vi "ReadData5.vi"() -> ()   [LabVIEW 2013]
uses:
  <vilib>/Utility/file.llb/Read From Spreadsheet File (DBL).vi
  <vilib>/Analysis/NI_AALPro.lvlib
  <vilib>/Analysis/NI_AALBase.lvlib
panel:
  out "Residual (V)":dbl format="%#_3g"
  in  "1st sweep":i32=400
  out "Peak Area Distribution":cluster{"Y":dbl[], "Y":dbl[]}[](graph)=[{"Y"=[nan, nan, nan, nan, nan, nan, nan, nan, nan, nan, nan, nan, nan, nan, nan, nan, nan, nan, nan, nan, nan, nan, nan, nan, nan, nan, nan, nan, nan, nan, nan, nan, nan, nan, nan, nan, nan, nan, nan, nan, nan, nan, nan, nan, nan, nan, nan, nan, nan, nan, nan, nan, nan, nan, nan, nan, nan, nan, nan, nan, nan, nan, nan, nan, nan, nan, nan, nan, nan, nan, nan, nan, nan, nan, nan, nan, nan, nan, nan, nan, nan, nan, nan, nan, nan, nan, nan, nan, nan, nan, nan, nan, nan, nan, nan, nan, nan, nan, nan, nan], "Y"=[0.0, 0.0, 0.0, 0.0, 0.0, 0.0, 0.0, 0.0, 0.0, 0.0, 0.0, 0.0, 0.0, 0.0, 0.0, 0.0, 0.0, 0.0, 0.0, 0.0, 0.0, 0.0, 0.0, 0.0, 0.0, 0.0, 0.0, 0.0, 0.0, 0.0, 0.0, 0.0, 0.0, 0.0, 0.0, 0.0, 0.0, 0.0, 0.0, 0.0, 0.0, 0.0, 0.0, 0.0, 0.0, 0.0, 0.0, 0.0, 0.0, 0.0, 0.0, 0.0, 0.0, 0.0, 0.0, 0.0, 0.0, 0.0, 0.0, 0.0, 0.0, 0.0, 0.0, 0.0, 0.0, 0.0, 0.0, 0.0, 0.0, 0.0, 0.0, 0.0, 0.0, 0.0, 0.0, 0.0, 0.0, 0.0, 0.0, 0.0, 0.0, 0.0, 0.0, 0.0, 0.0, 0.0, 0.0, 0.0, 0.0, 0.0, 0.0, 0.0, 0.0, 0.0, 0.0, 0.0, 0.0, 0.0, 0.0, 0.0]}]
  in  "# of sweeps":i32=500
  out "Mean Error":dbl=nan format="%#_2g"
  out "Mean Area":dbl=nan format="%#_4g"
  out "Peak Area":dbl(graph)=nan
  out "Spectrum #":i32=499
  out "Chars":i32=640716
  out "Fcen":dbl=213.0 format="%#_13g"
  in  "Fmin":dbl=212.8 format="%#_13g"
  in  "Fmax":dbl=213.2 format="%#_13g"
  out "# Data points":i32=81
  out "Peak Area (V-MHz)":dbl=nan format="%#_3g"
  out "Offset V":dbl=-0.006412499999999998 format="%#_3g"
  out "RMS Fit Error (V)":dbl=nan format="%#_2g"
  in  "Start sigma (V)":dbl=0.01 format="%#_13g"
  in  "Start offset (V)":dbl format="%#_13g"
  out "FWHM (MHz)":dbl=nan format="%#_3g"
  out "Center Freq (MHz)":dbl=nan
  out "Amplitude (V)":dbl=nan format="%#_3g"
  out "NMR Graph + Fit":cluster{cluster{dbl, "Numeric":dbl}[]}[](graph)
  out "File size (bytes)":i32=1284000
  out "File name":string="C:\\Documents and Settings\\Patrick McGaughey\\Desktop\\rssmt\\NMR3489061581.xls"
  # "Gaussian Fit Results"
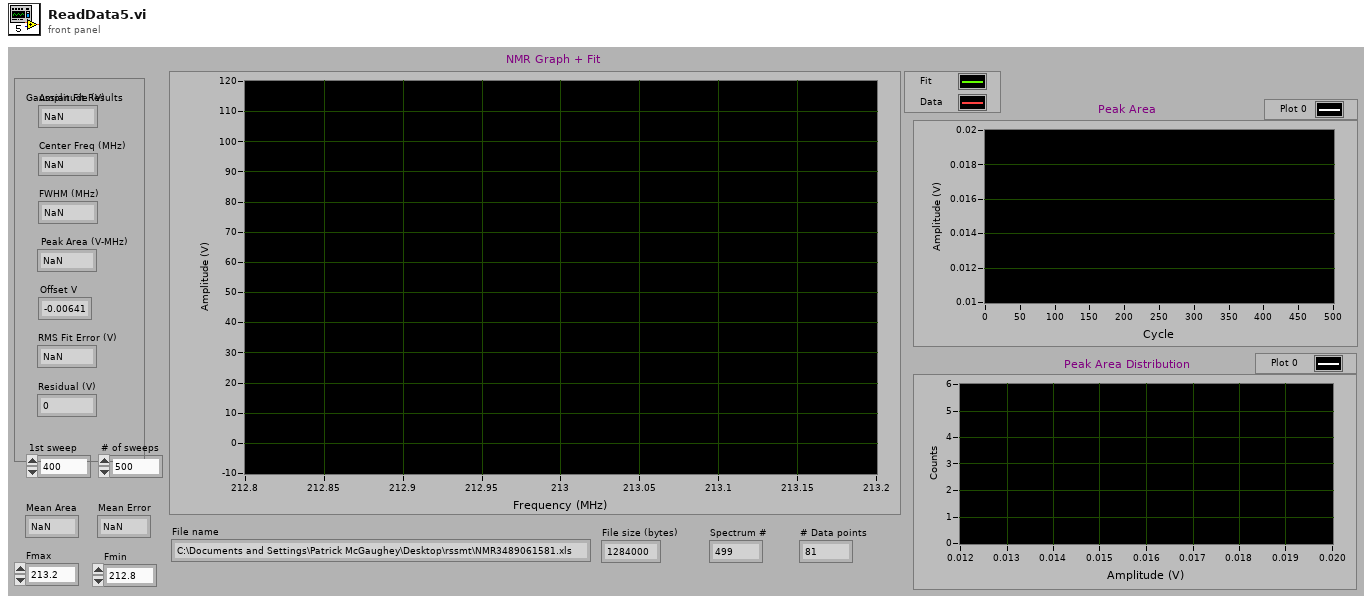
[diagram p1: front panel]
types:
  T1 = cluster{dbl, dbl, "Start sigma (V)":dbl, "Start offset (V)":dbl}
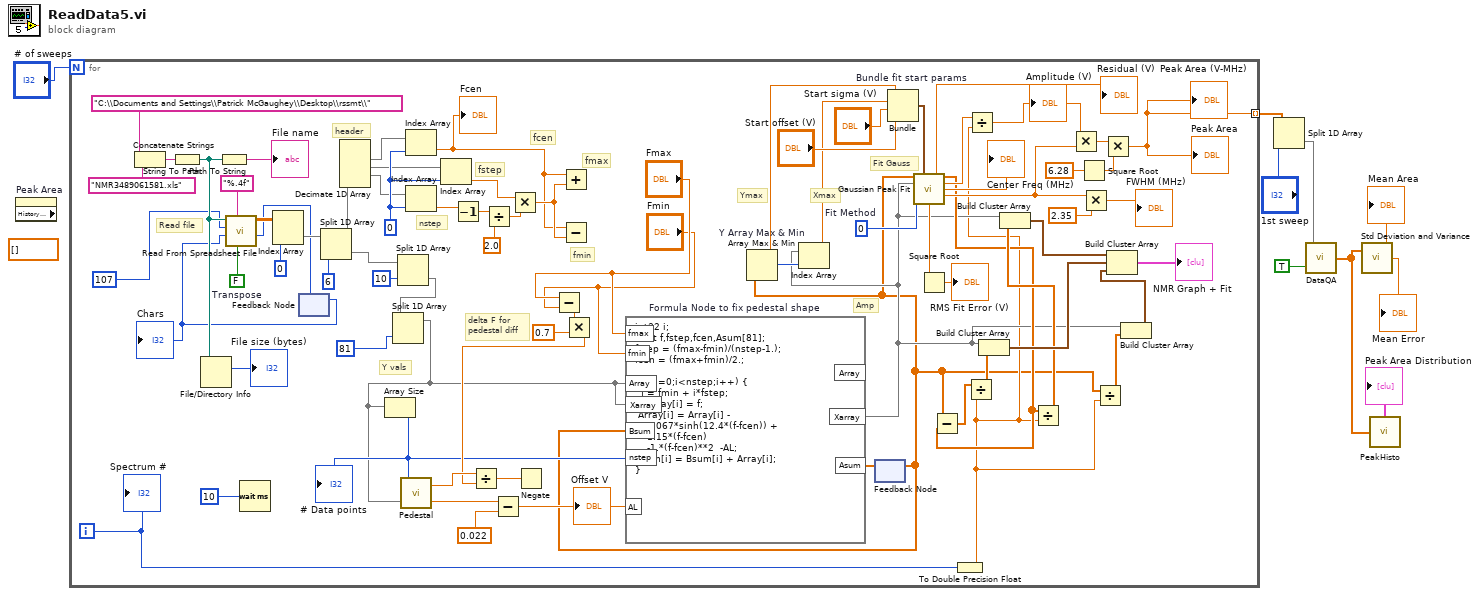
[diagram p0: block diagram]
diagram:
  (unwired) dbl[] []
  n1 = property on="Peak Area" class="WFChart (strict)" props=["History Data"]() -> ()  [unwired: 2 in, 3 out]
  n2 = for {
    N: "# of sweeps" -> [_]
    tunnel: [w36] -> w3 mode=indexing
    i -> [w27]
    w47 = 0
    w75 = 0  # Fit Method
    w83 = FALSE  # Transpose
    # "Fit Gauss"
    # "Read file"
    # "header"
    # "nstep"
    # "fstep"
    # "fcen"
    # "fmin"
    # "fmax"
    # "Amp"
    # "delta F for\npedestal diff"
    # "Ymax"
    # "Xmax"
    # "Y vals"
    n3 = Concatenate Strings "Concatenate Strings"("C:\\Documents and Settings\\Patrick McGaughey\\Desktop\\rssmt\\", "NMR3489061581.xls") -> (w86:string)
    n4 = String To Path(string=w86) -> (path=w82:path)
    n5 = File/Directory Info(path=w82) -> (size=→"File size (bytes)":i64)  [unwired: 1 in, 6 out]
    n6 = Path To String(path=w82) -> (string=→"File name":string)
    n7 = Wait (ms)(milliseconds to wait=10) -> ()  [unwired: 1 out]
    n8 = feedback #1() -> (w37:i32)  [unwired: 1 in]
    "Chars" <- w37
    n9 = call-poly <vilib>:"Read From Spreadsheet File.vi"("transpose (no:F)"=w83, "format (%.3f)"="%.4f", "start of read offset (chars.:0)"=w37, "number of rows (all:-1)"=107, "file path (dialog if empty)"=w82) -> ("mark after read (chars.)"=w38:i32, "all rows"=w55:dbl[][])  [unwired: 2 in, 3 out]
    n10 = Index Array "Index Array"(array=w55, index (col)=0) -> (element=w53:dbl[])  [unwired: 1 in]
    n11 = feedback-in #1(w38) -> ()
    n12 = Split 1D Array(array=w53, index=6) -> (first subarray=w56:dbl[], second subarray=w26:dbl[])
    n13 = Decimate 1D Array(w56) -> (w48:dbl[], w46:dbl[], w45:dbl[])  [unwired: 3 out]
    n14 = Split 1D Array(array=w26, index=10) -> (second subarray=w24:dbl[])  [unwired: 1 out]
    n15 = Split 1D Array(array=w24, index=81) -> (first subarray=w22:dbl[])  [unwired: 1 out]
    n16 = Array Size(array=w22) -> (size(s)=w58:i32)
    "# Data points" <- w58
    n17 = call "Pedestal.vi"("Varray"=w22, "ArraySize"=w58) -> ("Average"=w33:dbl, "L-R"=w69:dbl)
    n18 = Index Array "Index Array"(array=w48, index=w47) -> (element=w39:dbl)
    "Fcen" <- w39
    n19 = Index Array(array=w45, index=w47) -> (element=w43:dbl)
    n20 = Index Array(array=w46, index=w47) -> (element=w44:dbl)
    n21 = Decrement(x=w43) -> (x-1=w52:dbl)
    n22 = Divide(x=w52, y=2.0) -> (x/y=w50:dbl)
    n23 = Subtract(x=w33, y=0.022) -> (x-y=w32:dbl)
    "Offset V" <- w32
    n24 = Multiply(x=w44, y=w50) -> (x*y=w49:dbl)
    n25 = Subtract(x="Fmax", y="Fmin") -> (x-y=w67:dbl)
    n26 = Add(x=w39, y=w49) -> ()  [unwired: 1 out]
    n27 = Subtract(x=w39, y=w49) -> ()  [unwired: 1 out]
    n28 = Multiply(x=w67, y=0.7) -> (x*y=w66:dbl)
    n29 = Divide(x=w69, y=w66) -> (x/y=w65:dbl)
    n30 = Negate(x=w65) -> ()  [unwired: 1 out]
    n31 = feedback #2() -> (w10:dbl[])  [unwired: 1 in]
    n32 = formula code="int32 i;\nfloat f,fstep,fcen,Asum[81];\nfstep = (fmax-fmin)/(nstep-1.);\nfcen = (fmax+fmin)/2.;\n\nfor (i=0;i<nstep;i++) {\n  f = fmin + i*fstep;\n  Xarray[i] = f;\n Array[i] = Array[i] - \n    0.067*sinh(12.4*(f-fcen)) +\n    1.15*(f-fcen)  \n    -1.*(f-fcen)**2  -AL;\nAsum[i] = Bsum[i] + Array[i];\n}" "Formula Node to fix pedestal shape"("nstep"=w58, "fmin"="Fmin", "fmax"="Fmax", "AL"=w32, "Array"=w22, "Xarray"=w22, "Bsum"=w10) -> ("Xarray"=w14:dbl[], "Asum"=w31:dbl[])  [unwired: 1 out]
    n33 = Array Max & Min "Y Array Max & Min"(array=w10) -> (max value=w74:dbl, max index (indices)=w73:i32)  [unwired: 2 out]
    n34 = Index Array "Index Array"(array=w14, index=w73) -> (element=w62:dbl)
    n35 = feedback-in #2(w31) -> ()
    n36 = Bundle "Bundle fit start params"(w74, w62, "Start sigma (V)"="Start sigma (V)", "Start offset (V)"="Start offset (V)") -> (w78:T1)  [unwired: 1 in]
    n37 = call <vilib>:"Gaussian Peak Fit.vi"("Y"=w10, "initial guess"=w78, "X"=w14, "method"=w75) -> ("offset"=→"Residual (V)":dbl, "Best Gaussian Fit"=w15:dbl[], "amplitude"=w17:dbl, "center"=→"Center Freq (MHz)":dbl, "standard deviation"=w61:dbl, "residue"=w64:dbl)  [unwired: 5 in, 1 out]
    n38 = Square Root(x=w64) -> (sqrt(x)=→"RMS Fit Error (V)":dbl)
    n39 = Subtract(x=w10, y=w15) -> (x-y=w29:dbl[])
    n40 = To Double Precision Float(number=w27) -> (double precision float=w12:dbl)
    n41 = Divide(x=w29, y=w12) -> (x/y=w28:dbl[])
    n42 = Divide(x=w17, y=w12) -> (x/y=w16:dbl)
    "Amplitude (V)" <- w16
    n43 = Build Cluster Array ("Index & Bundle Cluster Array")(w14, w28) -> (w30:cluster{dbl, dbl}[])
    n44 = Divide(x=w15, y=w12) -> (x/y=w18:dbl[])
    n45 = Build Cluster Array ("Index & Bundle Cluster Array")(w14, w18) -> (w42:cluster{dbl, dbl}[])
    n46 = Multiply(x=w16, y=w61) -> (x*y=w70:dbl)
    n47 = Square Root(x=6.28) -> (sqrt(x)=w71:dbl)
    n48 = Multiply(x=w61, y=2.35) -> (x*y=→"FWHM (MHz)":dbl)
    n49 = Divide(x=w10, y=w12) -> (x/y=w11:dbl[])
    n50 = Multiply(x=w70, y=w71) -> (x*y=w36:dbl)
    "Peak Area (V-MHz)" <- w36
    "Peak Area" <- w36
    n51 = Build Cluster Array ("Index & Bundle Cluster Array")(w14, w11) -> (w13:cluster{dbl, dbl}[])
    n52 = Build Cluster Array "Build Cluster Array"(w42, w30, w13) -> (→"NMR Graph + Fit":cluster{cluster{dbl, dbl}[]}[])
    "Spectrum #" <- w27
  }
  n53 = Split 1D Array(array=w3, index="1st sweep") -> (second subarray=w1:dbl[])  [unwired: 1 out]
  n54 = call "DataQA.vi"("Quality cuts"=TRUE, "Data In"=w1) -> ("Data Out"=w4:dbl[])
  n55 = call <vilib>:"Std Deviation and Variance.vi"("X"=w4) -> ("mean"=→"Mean Area":dbl, "standard deviation"=→"Mean Error":dbl)  [unwired: 1 in, 1 out]
  n56 = call "PeakHisto.vi"("Data Out"=w4) -> ("XY Graph"=→"Peak Area Distribution":cluster{"Y":dbl[], "Y":dbl[]}[])
